vi "Do.vi"(8 "error in (no error)":errorcluster, 10 "Actor in":refnum<class "Actor.lvclass">, 11 "Update IODevInfo Msg in":refnum<class "Update IODevInfo Msg.lvclass">) -> (0 "error out":errorcluster, 2 "Actor out":refnum<class "Actor.lvclass">)   [LabVIEW 2015, in "Sequencer.lvlib" / "Update IODevInfo Msg.lvclass"]
doc: "(<B>Filename</B>: Actor Framework.lvlib:Message.lvclass:Do.vi)\n\nDefines what a message does when it is received by an actor. Generally, a message instructs an actor to invoke one of its methods. By default, this method does nothing. A child class must override it to define behavior. Create a child class by using the Actor Framework Message Maker dialog box."
uses:
  Update IODevInfo Msg.lvclass
  <vilib>/ActorFramework/Actor/Actor.lvclass
  Sequencer/Sequencer.lvclass
  Update IODevInfo Msg.lvclass/Update IODevInfo Msg.ctl
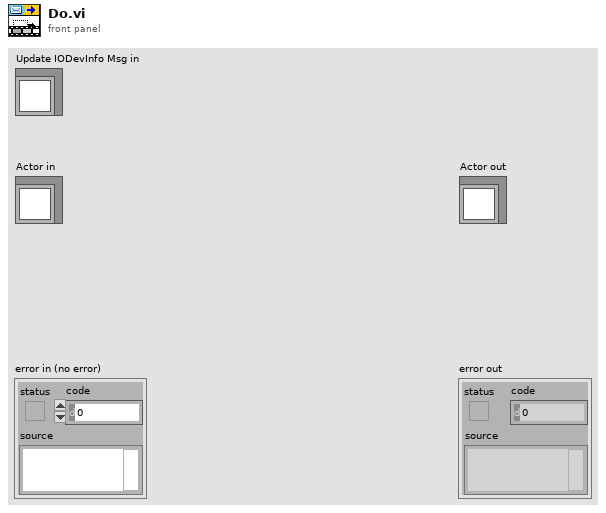
[diagram p1: front panel]
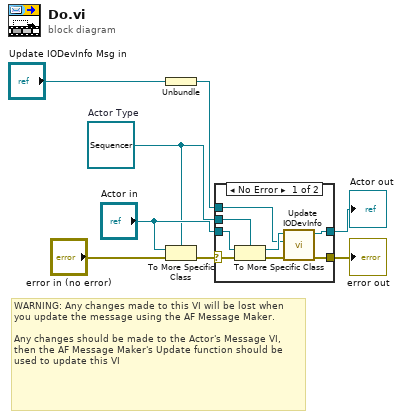
[diagram p0: block diagram]
diagram:
  w3 = refnum<class "Sequencer.lvclass"> refnum  # Actor Type
  # "WARNING: Any changes made to this VI will be lost when you update the message using the AF Message Maker.\n\nAny changes should be made to the Actor's Message VI, then the AF Message Maker's Update function should be used to update this VI"
  n1 = Unbundle("Update IODevInfo Msg in") -> (w2:refnum<class "IODevInfo.lvclass">)
  n2 = To More Specific Class(target class=w3, reference="Actor in", error in="error in (no error)") -> (error out=w7:errorcluster)  [unwired: 1 out]
  n3 = case shown="No Error" w7 {
    selector: w7 -> [w16 w18]
    tunnel: [w11 w18] -> w6
    tunnel: [w10 w17] -> w5
    tunnel: "Actor in" -> [w15 w17]
    tunnel: w3 -> [w14 _]
    tunnel: w2 -> [w9 _]
    frame No Error {
      n4 = To More Specific Class ("Actor Cast")(target class=w14, reference=w15, error in=w16) -> (specific class reference=w13:refnum<class "Sequencer.lvclass">, error out=w12:errorcluster)
      n5 = call "Update IODevInfo.vi"("error in (no error)"=w12, "IODevInfo"=w9, "Sequencer in"=w13) -> ("error out"=w11:errorcluster, "Sequencer out"=w10:refnum<class "Sequencer.lvclass">)  [unwired: 7 in]
    }
    frame Error {
    }
  }
  "error out" <- w6
  "Actor out" <- w5
